vi "Tester.vi"() -> ()   [LabVIEW 2012]
uses:
  Clear mode.ctl
  Shutter mode.ctl
  Trigger mode.ctl
panel:
  in  "temperature (°C)":i16
  out "Numeric":i32
  out "Image":T1(plugin-control)
  in  "stop":bool
  in  "Trigger mode":T2 items=["Timed", "Strobed", "Bulb", "Trigger first"]
  in  "Exposure (ms)":u32=30
  out "y size":u16
  out "x size":u16
  in  "EM gain":i16=3500
  in  "ADC gain":i16=1
  in  "# of clearing cycles":u16=1
  in  "Shutter mode":T3 items=["Never", "Pre-exposure", "Pre-sequence", "Pre-trigger"]
  in  "Clear mode":T4=1 items=["Never", "Pre-exposure", "Pre-sequence", "Post-sequence", "Pre- and post-sequence", "Pre-exp and post-seq"]
  out "error out":errorcluster
  in  "error in (no error)":errorcluster
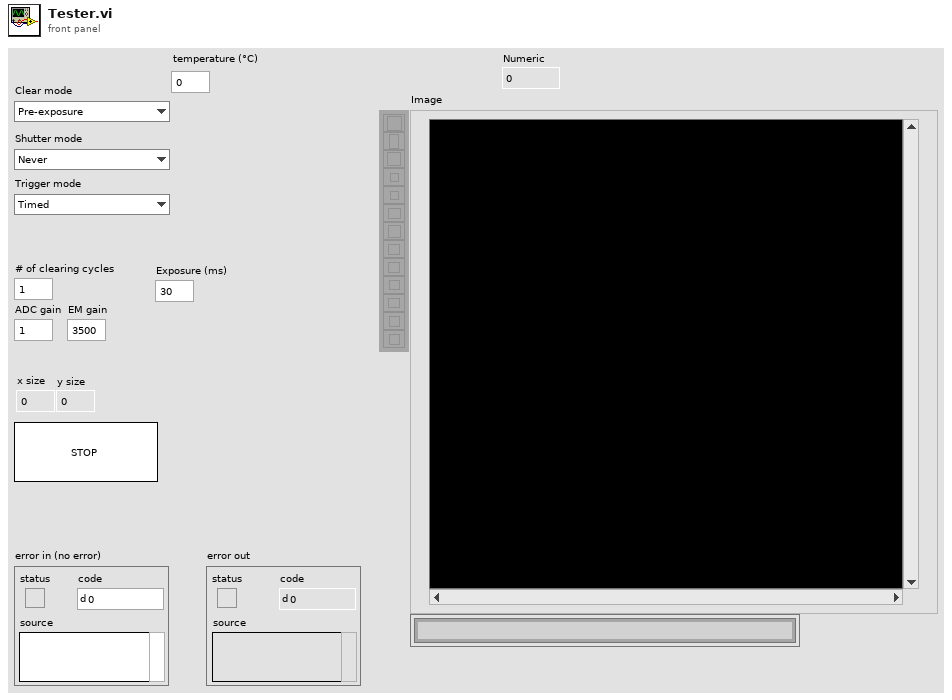
[diagram p1: front panel]
types:
  T1 = typedef "IMAQ Image.ctl" = refnum<image>
  T2 = typedef "Trigger mode.ctl" = i16
  T3 = typedef "Shutter mode.ctl" = i32
  T4 = typedef "Clear mode.ctl" = i32
  T5 = typedef "Image Type" = u32
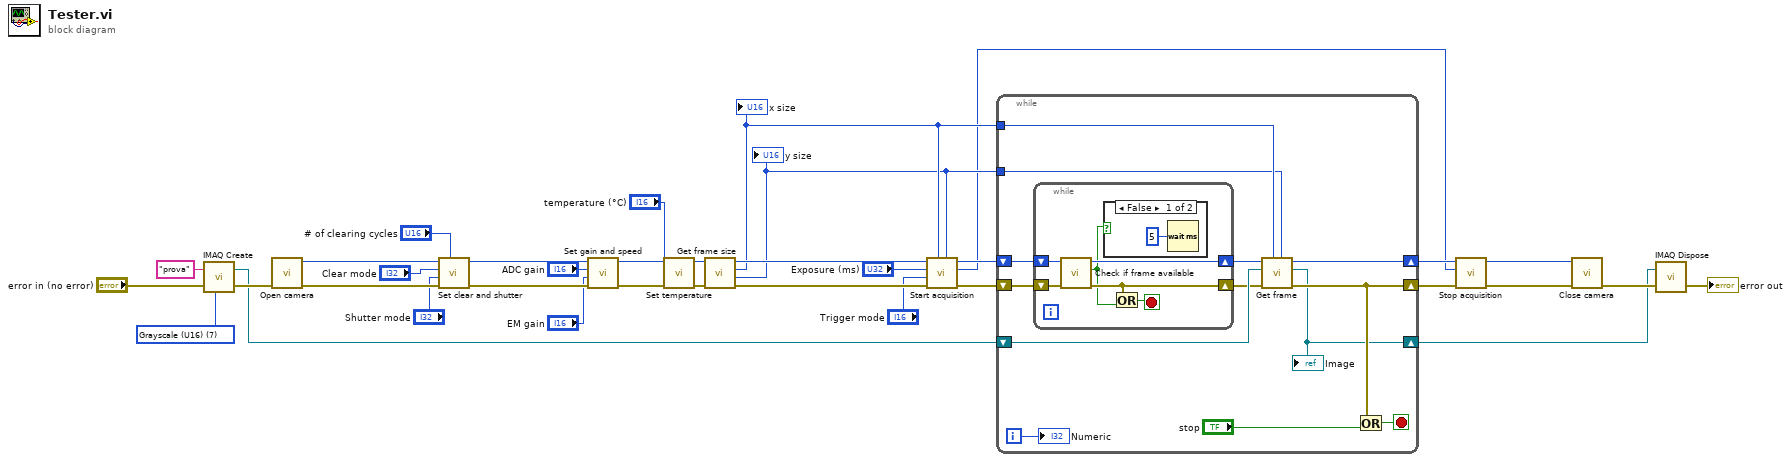
[diagram p0: block diagram]
diagram:
  w11 = T5 7 items=["Grayscale (U8)", "Grayscale (I16)", "Grayscale (SGL)", "Complex (CSG)", "RGB (U32)", "HSL (U32)", "RGB (U64)", "Grayscale (U16)"] ("Image Type")
  n1 = call "IMAQ Create"("Image Name"="prova", "Image Type"=w11, "error in (no error)"="error in (no error)") -> ("New Image"=w9:T1, "error out"=w12:errorcluster)  [unwired: 2 in]
  n2 = call "Open camera.vi"("error in"=w12) -> ("error out"=w33:errorcluster, "camera handle"=w31:i16)  [unwired: 9 in]
  n3 = call "Set clear and shutter.vi"("# of clearing cycles"="# of clearing cycles", "error in (no error)"=w33, "Shutter mode"="Shutter mode", "Clear mode"="Clear mode", "camera handle in"=w31) -> ("error out"=w34:errorcluster, "camera handle out"=w30:i16)  [unwired: 5 in]
  n4 = call "Set gain and speed.vi"("error in (no error)"=w34, "EM gain"="EM gain", "ADC gain"="ADC gain", "camera handle in"=w30) -> ("error out"=w3:errorcluster, "camera handle out"=w5:i16)  [unwired: 6 in]
  n5 = call "Set temperature.vi"("error in (no error)"=w3, "temperature (°C)"="temperature (°C)", "camera handle in"=w5) -> ("error out"=w2:errorcluster, "camera handle out"=w4:i16)  [unwired: 7 in]
  n6 = call "Get frame size.vi"("error in (no error)"=w2, "camera handle in"=w4) -> ("error out"=w23:errorcluster, "y size"=w13:u16, "x size"=w14:u16, "camera handle out"=w24:i16)  [unwired: 6 in]
  "x size" <- w14
  "y size" <- w13
  n7 = call "Start acquisition.vi"("y frame size"=w13, "x frame size"=w14, "error in (no error)"=w23, "Trigger mode"="Trigger mode", "Exposure"="Exposure (ms)", "camera handle in"=w24) -> ("error out"=w20:errorcluster, "buffer ref out"=w6:i32, "camera handle out"=w19:i16)  [unwired: 3 in]
  n8 = while {
    shift-right: [w46] -> w17
    shift-left: w20 -> [w40]
    shift-right: [w48] -> w18
    shift-left: w19 -> [w39]
    tunnel: w14 -> [w44]
    tunnel: w13 -> [w43]
    shift-right: [w41] -> w7
    shift-left: w9 -> [w42]
    i -> [w36]
    stop <- w45 stop-if-true
    n9 = while {
      shift-right: [w51] -> w37
      shift-left: w40 -> [w54]
      shift-right: [w52] -> w38
      shift-left: w39 -> [w53]
      stop <- w49 stop-if-true
      n10 = call "Check if frame available.vi"("error in (no error)"=w54, "camera handle in"=w53) -> ("error out"=w51:errorcluster, "is frame ready?"=w50:bool, "camera handle out"=w52:i16)  [unwired: 7 in]
      n11 = case shown="False" w50 {
        frame False {
          n12 = Wait (ms)(milliseconds to wait=u32 5) -> ()  [unwired: 1 out]
        }
        frame True {
        }
      }
      n13 = Or(x=w51, y=w50) -> (x .or. y?=w49:bool)
    }
    n14 = call "Get frame.vi"("frame y size"=w43, "frame x size"=w44, "error in (no error)"=w37, "Image in"=w42, "camera handle in"=w38) -> ("error out"=w46:errorcluster, "Image out"=w41:T1, "camera handle out"=w48:i16)  [unwired: 4 in]
    "Image" <- w41
    n15 = Or(x=w46, y="stop") -> (x .or. y?=w45:bool)
    "Numeric" <- w36
  }
  n16 = call "Stop acquisition.vi"("error in (no error)"=w17, "buffer ref"=w6, "camera handle in"=w18) -> ("error out"=w15:errorcluster, "camera handle out"=w16:i16)  [unwired: 7 in]
  n17 = call "Close camera.vi"("error in (no error)"=w15, "camera handle in"=w16) -> ("error out"=w35:errorcluster)  [unwired: 9 in]
  n18 = call "IMAQ Dispose"("Image"=w7, "error in (no error)"=w35) -> ("error out"=→"error out":errorcluster)  [unwired: 4 in]
